vi "Weather Parse Test.vi"() -> ()   [LabVIEW 2020, in "CDM-Config.lvlib"] (continued)
\"Avoid\",\n                \"parameters\": {\n                    \"AWIPSidentifier\": [\n                        \"MWWCLE\"\n                    ],\n                    \"WMOidentifier\": [\n                        \"WHUS71 KCLE 031442\"\n                    ],\n                    \"NWSheadline\": [\n                        \"SMALL CRAFT ADVISORY REMAINS IN EFFECT UNTIL 7 PM EST THURSDAY... ...LOW WATER ADVISORY REMAINS IN EFFECT UNTIL 10 PM EST THIS EVENING\"\n                    ],\n                    \"BLOCKCHANNEL\": [\n                        \"EAS\",\n                        \"NWEM\",\n                        \"CMAS\"\n                    ],\n                    \"VTEC\": [\n                        \"/O.CON.KCLE.SC.Y.0072.000000T0000Z-251205T0000Z/\"\n                    ],\n                    \"eventEndingTime\": [\n                        \"2025-12-04T19:00:00-05:00\"\n                    ],\n                    \"expiredReferences\": [\n                        \"w-nws.webmaster@noaa.gov,urn:oid:2.49.0.1.840.0.0c886383843e06dfcc6ba0a1dce77e56032b6216.002.1,2025-12-02T21:44:00-05:00\"\n                    ]\n                },\n                \"scope\": \"Public\",\n                \"code\": \"IPAWSv1.0\",\n                \"language\": \"en-US\",\n                \"web\": \"http://www.weather.gov\",\n                \"eventCode\": {\n                    \"SAME\": [\n                        \"NWS\"\n                    ],\n                    \"NationalWeatherService\": [\n                        \"SCY\"\n                    ]\n                }\n            }\n        },\n        {\n            \"id\": \"https://api.weather.gov/alerts/urn:oid:2.49.0.1.840.0.459139686b06dc7377a32ee0b95bac1f049c2e93.001.1\",\n            \"type\": \"Feature\",\n            \"geometry\": null,\n            \"properties\": {\n                \"@id\": \"https://api.weather.gov/alerts/urn:oid:2.49.0.1.840.0.459139686b06dc7377a32ee0b95bac1f049c2e93.001.1\",\n                \"@type\": \"wx:Alert\",\n                \"id\": \"urn:oid:2.49.0.1.840.0.459139686b06dc7377a32ee0b95bac1f049c2e93.001.1\",\n                \"areaDesc\": \"Eastern Glacier, Western Toole, and Central Pondera; Southern High Plains; Eastern Pondera and Eastern Teton; Cascade County below 5000ft; Judith Basin County and Judith Gap; Gates of the Mountains\",\n                \"geocode\": {\n                    \"SAME\": [\n                        \"030035\",\n                        \"030073\",\n                        \"030101\",\n                        \"030049\",\n                        \"030099\",\n                        \"030013\",\n                        \"030045\",\n                        \"030027\"\n                    ],\n                    \"UGC\": [\n                        \"MTZ303\",\n                        \"MTZ308\",\n                        \"MTZ309\",\n                        \"MTZ312\",\n                        \"MTZ313\",\n                        \"MTZ316\"\n                    ]\n                },\n                \"affectedZones\": [\n                    \"https://api.weather.gov/zones/forecast/MTZ303\",\n                    \"https://api.weather.gov/zones/forecast/MTZ308\",\n                    \"https://api.weather.gov/zones/forecast/MTZ309\",\n                    \"https://api.weather.gov/zones/forecast/MTZ312\",\n                    \"https://api.weather.gov/zones/forecast/MTZ313\",\n                    \"https://api.weather.gov/zones/forecast/MTZ316\"\n                ],\n                \"references\": [],\n                \"sent\": \"2025-12-03T07:40:00-07:00\",\n                \"effective\": \"2025-12-03T07:40:00-07:00\",\n                \"onset\": \"2025-12-03T07:40:00-07:00\",\n                \"expires\": \"2025-12-03T10:00:00-07:00\",\n                \"ends\": null,\n                \"status\": \"Actual\",\n                \"messageType\": \"Alert\",\n                \"category\": \"Met\",\n                \"severity\": \"Moderate\",\n                \"certainty\": \"Observed\",\n                \"urgency\": \"Expected\",\n                \"event\": \"Special Weather Statement\",\n                \"sender\": \"w-nws.webmaster@noaa.gov\",\n                \"senderName\": \"NWS Great Falls MT\",\n                \"headline\": \"Special Weather Statement issued December 3 at 7:40AM MST by NWS Great Falls MT\",\n                \"description\": \"Patchy dense freezing fog is possible across portions of north-\\ncentral Montana this morning. Reduced visibility, in combination\\nwith icy roads, may make travel difficult at times. Motorists\\nshould be prepared for sudden changes in visibility and road\\nconditions.\",\n                \"instruction\": null,\n                \"response\": \"Execute\",\n                \"parameters\": {\n                    \"AWIPSidentifier\": [\n                        \"SPSTFX\"\n                    ],\n                    \"WMOidentifier\": [\n                        \"WWUS85 KTFX 031440\"\n                    ],\n                    \"BLOCKCHANNEL\": [\n                        \"EAS\",\n                        \"NWEM\",\n                        \"CMAS\"\n                    ],\n                    \"EAS-ORG\": [\n                        \"WXR\"\n                    ]\n                },\n                \"scope\": \"Public\",\n                \"code\": \"IPAWSv1.0\",\n                \"language\": \"en-US\",\n                \"web\": \"http://www.weather.gov\",\n                \"eventCode\": {\n                    \"SAME\": [\n                        \"SPS\"\n                    ],\n                    \"NationalWeatherService\": [\n                        \"SPS\"\n                    ]\n                }\n            }\n        },\n        {\n            \"id\": \"https://api.weather.gov/alerts/urn:oid:2.49.0.1.840.0.d9de63c9900d21dbac134cf2fe7828d3f5276171.002.2\",\n            \"type\": \"Feature\",\n            \"geometry\": null,\n            \"properties\": {\n                \"@id\": \"https://api.weather.gov/alerts/urn:oid:2.49.0.1.840.0.d9de63c9900d21dbac134cf2fe7828d3f5276171.002.2\",\n                \"@type\": \"wx:Alert\",\n                \"id\": \"urn:oid:2.49.0.1.840.0.d9de63c9900d21dbac134cf2fe7828d3f5276171.002.2\",\n                \"areaDesc\": \"Penobscot Bay; Casco Bay\",\n                \"geocode\": {\n                    \"SAME\": [\n                        \"073151\",\n                        \"073153\"\n                    ],\n                    \"UGC\": [\n                        \"ANZ151\",\n                        \"ANZ153\"\n                    ]\n                },\n                \"affectedZones\": [\n                    \"https://api.weather.gov/zones/forecast/ANZ151\",\n                    \"https://api.weather.gov/zones/forecast/ANZ153\"\n                ],\n                \"references\": [],\n                \"sent\": \"2025-12-03T09:35:00-05:00\",\n                \"effective\": \"2025-12-03T09:35:00-05:00\",\n                \"onset\": \"2025-12-04T13:00:00-05:00\",\n                \"expires\": \"2025-12-03T23:45:00-05:00\",\n                \"ends\": \"2025-12-05T07:00:00-05:00\",\n                \"status\": \"Actual\",\n                \"messageType\": \"Alert\",\n                \"category\": \"Met\",\n                \"severity\": \"Minor\",\n                \"certainty\": \"Likely\",\n                \"urgency\": \"Expected\",\n                \"event\": \"Small Craft Advisory\",\n                \"sender\": \"w-nws.webmaster@noaa.gov\",\n                \"senderName\": \"NWS Gray ME\",\n                \"headline\": \"Small Craft Advisory issued December 3 at 9:35AM EST until December 5 at 7:00AM EST by NWS Gray ME\",\n                \"description\": \"* WHAT...Northwest winds 15 to 25 kt with gusts up to 30 kt and\\nseas 2 to 5 ft expected.\\n\\n* WHERE...Penobscot Bay and Casco Bay.\\n\\n* WHEN...From 1 PM Thursday to 7 AM EST Friday.\\n\\n* IMPACTS...Conditions will be hazardous to small craft.\",\n                \"instruction\": \"Inexperienced mariners, especially those operating smaller\\nvessels, should avoid navigating in hazardous conditions.\",\n                \"response\": \"Avoid\",\n                \"parameters\": {\n                    \"AWIPSidentifier\": [\n                        \"MWWGYX\"\n                    ],\n                    \"WMOidentifier\": [\n                        \"WHUS71 KGYX 031435\"\n                    ],\n                    \"NWSheadline\": [\n                        \"SMALL CRAFT ADVISORY IN EFFECT FROM 1 PM THURSDAY TO 7 AM EST FRIDAY... ...SMALL CRAFT ADVISORY IS CANCELLED\"\n                    ],\n                    \"BLOCKCHANNEL\": [\n                        \"EAS\",\n                        \"NWEM\",\n                        \"CMAS\"\n                    ],\n                    \"VTEC\": [\n                        \"/O.NEW.KGYX.SC.Y.0091.251204T1800Z-251205T1200Z/\"\n                    ],\n                    \"eventEndingTime\": [\n                        \"2025-12-05T07:00:00-05:00\"\n                    ]\n                },\n                \"scope\": \"Public\",\n                \"code\": \"IPAWSv1.0\",\n                \"language\": \"en-US\",\n                \"web\": \"http://www.weather.gov\",\n                \"eventCode\": {\n                    \"SAME\": [\n                        \"NWS\"\n                    ],\n                    \"NationalWeatherService\": [\n                        \"SCY\"\n                    ]\n                }\n            }\n        },\n        {\n            \"id\": \"https://api.weather.gov/alerts/urn:oid:2.49.0.1.840.0.d9de63c9900d21dbac134cf2fe7828d3f5276171.001.2\",\n            \"type\": \"Feature\",\n            \"geometry\": null,\n            \"properties\": {\n                \"@id\": \"https://api.weather.gov/alerts/urn:oid:2.49.0.1.840.0.d9de63c9900d21dbac134cf2fe7828d3f5276171.001.2\",\n                \"@type\": \"wx:Alert\",\n                \"id\": \"urn:oid:2.49.0.1.840.0.d9de63c9900d21dbac134cf2fe7828d3f5276171.001.2\",\n                \"areaDesc\": \"Coastal Waters from Stonington, ME to Port Clyde, ME out 25 NM; Coastal Waters from Port Clyde, ME to Cape Elizabeth, ME out 25 NM; Coastal Waters from Cape Elizabeth, ME to Merrimack River, MA out 25 NM\",\n                \"geocode\": {\n                    \"SAME\": [\n                        \"073150\",\n                        \"073152\",\n                        \"073154\"\n                    ],\n                    \"UGC\": [\n                        \"ANZ150\",\n                        \"ANZ152\",\n                        \"ANZ154\"\n                    ]\n                },\n                \"affectedZones\": [\n                    \"https://api.weather.gov/zones/forecast/ANZ150\",\n                    \"https://api.weather.gov/zones/forecast/ANZ152\",\n                    \"https://api.weather.gov/zones/forecast/ANZ154\"\n                ],\n                \"references\": [],\n                \"sent\": \"2025-12-03T09:35:00-05:00\",\n                \"effective\": \"2025-12-03T09:35:00-05:00\",\n                \"onset\": \"2025-12-04T15:00:00-05:00\",\n                \"expires\": \"2025-12-03T23:45:00-05:00\",\n                \"ends\": \"2025-12-05T00:00:00-05:00\",\n                \"status\": \"Actual\",\n                \"messageType\": \"Alert\",\n                \"category\": \"Met\",\n                \"severity\": \"Moderate\",\n                \"certainty\": \"Likely\",\n                \"urgency\": \"Expected\",\n                \"event\": \"Gale Warning\",\n                \"sender\": \"w-nws.webmaster@noaa.gov\",\n                \"senderName\": \"NWS Gray ME\",\n                \"headline\": \"Gale Warning issued December 3 at 9:35AM EST until December 5 at 12:00AM EST by NWS Gray ME\",\n                \"description\": \"* WHAT...Northwest winds 20 to 30 kt with gusts up to 40 kt and\\nseas 5 to 8 ft expected.\\n\\n* WHERE...Coastal Waters from Stonington, ME to Port Clyde, ME\\nout 25 NM, Coastal Waters from Port Clyde, ME to Cape\\nElizabeth, ME out 25 NM and Coastal Waters from Cape\\nElizabeth, ME to Merrimack River, MA out 25 NM.\\n\\n* WHEN...From 3 PM Thursday to midnight EST Thursday night.\\n\\n* IMPACTS...Strong winds will cause hazardous seas which could\\ncapsize or damage vessels and reduce visibility.\",\n                \"instruction\": \"Mariners should alter plans to avoid these hazardous conditions.\\nRemain in port, seek safe harbor, alter course, and/or secure the\\nvessel for severe conditions.\",\n                \"response\": \"Avoid\",\n                \"parameters\": {\n                    \"AWIPSidentifier\": [\n                        \"MWWGYX\"\n                    ],\n                    \"WMOidentifier\": [\n                        \"WHUS71 KGYX 031435\"\n                    ],\n                    \"NWSheadline\": [\n                        \"GALE WARNING IN EFFECT FROM 3 PM THURSDAY TO MIDNIGHT EST THURSDAY NIGHT... ...GALE WARNING IS CANCELLED\"\n                    ],\n                    \"BLOCKCHANNEL\": [\n                        \"EAS\",\n                        \"NWEM\",\n                        \"CMAS\"\n                    ],\n                    \"VTEC\": [\n                        \"/O.NEW.KGYX.GL.W.0036.251204T2000Z-251205T0500Z/\"\n                    ],\n                    \"eventEndingTime\": [\n                        \"2025-12-05T00:00:00-05:00\"\n                    ]\n                },\n                \"scope\": \"Public\",\n                \"code\": \"IPAWSv1.0\",\n                \"language\": \"en-US\",\n                \"web\": \"http://www.weather.gov\",\n                \"eventCode\": {\n                    \"SAME\": [\n                        \"NWS\"\n                    ],\n                    \"NationalWeatherService\": [\n                        \"GLW\"\n                    ]\n                }\n            }\n        },\n        {\n            \"id\": \"https://api.weather.gov/alerts/urn:oid:2.49.0.1.840.0.168ce73ea8a3865ae0fef26c6698f44454ec2ed2.001.1\",\n            \"type\": \"Feature\",\n            \"geometry\": null,\n            \"properties\": {\n                \"@id\": \"https://api.weather.gov/alerts/urn:oid:2.49.0.1.840.0.168ce73ea8a3865ae0fef26c6698f44454ec2ed2.001.1\",\n                \"@type\": \"wx:Alert\",\n                \"id\": \"urn:oid:2.49.0.1.840.0.168ce73ea8a3865ae0fef26c6698f44454ec2ed2.001.1\",\n                \"areaDesc\": \"St Joseph to South Haven MI; South Haven to Holland MI; Holland to Grand Haven MI; Grand Haven to Whitehall MI; Whitehall to Pentwater MI; Pentwater to Manistee MI\",\n                \"geocode\": {\n                    \"SAME\": [\n                        \"092844\",\n                        \"092845\",\n                        \"092846\",\n                        \"092847\",\n                        \"092848\",\n                        \"092849\"\n                    ],\n                    \"UGC\": [\n                        \"LMZ844\",\n                        \"LMZ845\",\n                        \"LMZ846\",\n                        \"LMZ847\",\n                        \"LMZ848\",\n                        \"LMZ849\"\n                    ]\n                },\n                \"affectedZones\": [\n                    \"https://api.weather.gov/zones/forecast/LMZ844\",\n                    \"https://api.weather.gov/zones/forecast/LMZ845\",\n                    \"https://api.weather.gov/zones/forecast/LMZ846\",\n                    \"https://api.weather.gov/zones/forecast/LMZ847\",\n                    \"https://api.weather.gov/zones/forecast/LMZ848\",\n                    \"https://api.weather.gov/zones/forecast/LMZ849\"\n                ],\n                \"references\": [\n                    {\n                        \"@id\": \"https://api.weather.gov/alerts/urn:oid:2.49.0.1.840.0.7aaab00944e439757f97bf60c2973af97298ac0f.001.1\",\n                        \"identifier\": \"urn:oid:2.49.0.1.840.0.7aaab00944e439757f97bf60c2973af97298ac0f.001.1\",\n                        \"sender\": \"w-nws.webmaster@noaa.gov\",\n                        \"sent\": \"2025-12-03T03:29:00-05:00\"\n                    }\n                ],\n                \"sent\": \"2025-12-03T09:32:00-05:00\",\n                \"effective\": \"2025-12-03T09:32:00-05:00\",\n                \"onset\": \"2025-12-03T09:32:00-05:00\",\n                \"expires\": \"2025-12-03T17:45:00-05:00\",\n                \"ends\": \"2025-12-04T19:00:00-05:00\",\n                \"status\": \"Actual\",\n                \"messageType\": \"Update\",\n                \"category\": \"Met\",\n                \"severity\": \"Minor\",\n                \"certainty\": \"Likely\",\n                \"urgency\": \"Expected\",\n                \"event\": \"Small Craft Advisory\",\n                \"sender\": \"w-nws.webmaster@noaa.gov\",\n                \"senderName\": \"NWS Grand Rapids MI\",\n                \"headline\": \"Small Craft Advisory issued December 3 at 9:32AM EST until December 4 at 7:00PM EST by NWS Grand Rapids MI\",\n                \"description\": \"* WHAT...Northwest winds 15 to 25 knots with gusts up to 30\\nknots and waves 6 to 9 feet.\\n\\n* WHERE...St Joseph to Manistee.\\n\\n* WHEN...Until 7 PM EST Thursday.\\n\\n* IMPACTS...Conditions will be hazardous to small craft.\",\n                \"instruction\": \"Inexperienced mariners, especially those operating smaller\\nvessels, should avoid navigating in hazardous conditions.\",\n                \"response\": \"Avoid\",\n                \"parameters\": {\n                    \"AWIPSidentifier\": [\n                        \"MWWGRR\"\n                    ],\n                    \"WMOidentifier\": [\n                        \"WHUS73 KGRR 031432\"\n                    ],\n                    \"NWSheadline\": [\n                        \"SMALL CRAFT ADVISORY REMAINS IN EFFECT UNTIL 7 PM EST THURSDAY\"\n                    ],\n                    \"BLOCKCHANNEL\": [\n                        \"EAS\",\n                        \"NWEM\",\n                        \"CMAS\"\n                    ],\n                    \"VTEC\": [\n                        \"/O.CON.KGRR.SC.Y.0105.000000T0000Z-251205T0000Z/\"\n                    ],\n                    \"eventEndingTime\": [\n                        \"2025-12-04T19:00:00-05:00\"\n                    ],\n                    \"expiredReferences\": [\n                        \"w-nws.webmaster@noaa.gov,urn:oid:2.49.0.1.840.0.d51c6ec7dcdb20057f5ceabbc87dc36d93f53d9d.001.1,2025-12-02T22:57:00-05:00 w-nws.webmaster@noaa.gov,urn:oid:2.49.0.1.840.0.37bcc3e39a4ce8355e137c1eb2919fee8e6cd4f1.001.1,2025-12-02T15:51:00-05:00 w-nws.webmaster@noaa.gov,urn:oid:2.49.0.1.840.0.c3d7b241827877fcb2062e6796861e8d3cd92a63.001.1,2025-12-02T09:46:00-05:00 w-nws.webmaster@noaa.gov,urn:oid:2.49.0.1.840.0.67f802fa2a1d1ee3a1aa8fcbfdeb00afe1d79cbe.001.1,2025-12-02T03:07:00-05:00\"\n                    ]\n                },\n                \"scope\": \"Public\",\n                \"code\": \"IPAWSv1.0\",\n                \"language\": \"en-US\",\n                \"web\": \"http://www.weather.gov\",\n                \"eventCode\": {\n                    \"SAME\": [\n                        \"NWS\"\n                    ],\n                    \"NationalWeatherService\": [\n                        \"SCY\"\n                    ]\n                }\n            }\n        },\n        {\n            \"id\": \"https://api.weather.gov/alerts/urn:oid:2.49.0.1.840.0.1012c94d5f34968dad73e0ece48bd6552b3e5229.005.1\",\n            \"type\": \"Feature\",\n            \"geometry\": null,\n            \"properties\": {\n                \"@id\": \"https://api.weather.gov/alerts/urn:oid:2.49.0.1.840.0.1012c94d5f34968dad73e0ece48bd6552b3e5229.005.1\",\n                \"@type\": \"wx:Alert\",\n                \"id\": \"urn:oid:2.49.0.1.840.0.1012c94d5f34968dad73e0ece48bd6552b3e5229.005.1\",\n                \"areaDesc\": \"Boston Harbor; Narragansett Bay\",\n                \"geocode\": {\n                    \"SAME\": [\n                        \"073230\",\n                        \"073236\"\n                    ],\n                    \"UGC\": [\n                        \"ANZ230\",\n                        \"ANZ236\"\n                    ]\n                },\n                \"affectedZones\": [\n                    \"https://api.weather.gov/zones/forecast/ANZ230\",\n                    \"https://api.weather.gov/zones/forecast/ANZ236\"\n                ],\n                \"references\": [],\n                \"sent\": \"2025-12-03T09:03:00-05:00\",\n                \"effective\": \"2025-12-03T09:03:00-05:00\",\n                \"onset\": \"2025-12-04T13:00:00-05:00\",\n                \"expires\": \"2025-12-03T22:15:00-05:00\",\n                \"ends\": \"2025-12-05T01:00:00-05:00\",\n                \"status\": \"Actual\",\n                \"messageType\": \"Alert\",\n                \"category\": \"Met\",\n                \"severity\": \"Moderate\",\n                \"certainty\": \"Possible\",\n                \"urgency\": \"Future\",\n                \"event\": \"Gale Watch\",\n                \"sender\": \"w-nws.webmaster@noaa.gov\",\n                \"senderName\": \"NWS Boston/Norton MA\",\n                \"headline\": \"Gale Watch issued December 3 at 9:03AM EST until December 5 at 1:00AM EST by NWS Boston/Norton MA\",\n                \"description\": \"* WHAT...Northwest winds 15 to 25 kt with gusts up to 35 kt and\\nwaves 2 to 3 feet possible.\\n\\n* WHERE...In Massachusetts coastal waters, Boston Harbor. In\\nRhode Island coastal waters, Narragansett Bay.\\n\\n* WHEN...From Thursday afternoon through late Thursday night.\\n\\n* IMPACTS...Strong winds can cause hazardous waves which could\\ncapsize or damage vessels and reduce visibility.\",\n                \"instruction\": \"Mariners should consider altering plans to avoid possible\\nhazardous conditions.  Remain in port, seek safe harbor, alter\\ncourse, and/or secure the vessel for severe wind and seas.\",\n                \"response\": \"Prepare\",\n                \"parameters\": {\n                    \"AWIPSidentifier\": [\n                        \"MWWBOX\"\n                    ],\n                    \"WMOidentifier\": [\n                        \"WHUS71 KBOX 031403\"\n                    ],\n                    \"NWSheadline\": [\n                        \"GALE WATCH IN EFFECT FROM THURSDAY AFTERNOON THROUGH LATE THURSDAY NIGHT\"\n                    ],\n                    \"BLOCKCHANNEL\": [\n                        \"EAS\",\n                        \"NWEM\",\n                        \"CMAS\"\n                    ],\n                    \"VTEC\": [\n                        \"/O.NEW.KBOX.GL.A.0024.251204T1800Z-251205T0600Z/\"\n                    ],\n                    \"eventEndingTime\": [\n                        \"2025-12-05T01:00:00-05:00\"\n                    ]\n                },\n                \"scope\": \"Public\",\n                \"code\": \"IPAWSv1.0\",\n                \"language\": \"en-US\",\n                \"web\": \"http://www.weather.gov\",\n                \"eventCode\": {\n                    \"SAME\": [\n                        \"NWS\"\n                    ],\n                    \"NationalWeatherService\": [\n                        \"GLA\"\n                    ]\n                }\n            }\n        },\n        {\n            \"id\": \"https://api.weather.gov/alerts/urn:oid:2.49.0.1.840.0.1012c94d5f34968dad73e0ece48bd6552b3e5229.001.3\",\n            \"type\": \"Feature\",\n            \"geometry\": null,\n            \"properties\": {\n                \"@id\": \"https://api.weather.gov/alerts/urn:oid:2.49.0.1.840.0.1012c94d5f34968dad73e0ece48bd6552b3e5229.001.3\",\n                \"@type\": \"wx:Alert\",\n                \"id\": \"urn:oid:2.49.0.1.840.0.1012c94d5f34968dad73e0ece48bd6552b3e5229.001.3\",\n                \"areaDesc\": \"Coastal waters east of Ipswich Bay and the Stellwagen Bank National Marine Sanctuary; Coastal waters from Provincetown MA to Chatham MA to Nantucket MA out 20 nm; Coastal Waters extending out to 25 nm South of Marthas Vineyard and Nantucket\",\n                \"geocode\": {\n                    \"SAME\": [\n                        \"073250\",\n                        \"073254\",\n                        \"073255\"\n                    ],\n                    \"UGC\": [\n                        \"ANZ250\",\n                        \"ANZ254\",\n                        \"ANZ255\"\n                    ]\n                },\n                \"affectedZones\": [\n                    \"https://api.weather.gov/zones/forecast/ANZ250\",\n                    \"https://api.weather.gov/zones/forecast/ANZ254\",\n                    \"https://api.weather.gov/zones/forecast/ANZ255\"\n                ],\n                \"references\": [],\n                \"sent\": \"2025-12-03T09:03:00-05:00\",\n                \"effective\": \"2025-12-03T09:03:00-05:00\",\n                \"onset\": \"2025-12-04T13:00:00-05:00\",\n                \"expires\": \"2025-12-03T22:15:00-05:00\",\n                \"ends\": \"2025-12-05T04:00:00-05:00\",\n                \"status\": \"Actual\",\n                \"messageType\": \"Alert\",\n                \"category\": \"Met\",\n                \"severity\": \"Moderate\",\n                \"certainty\": \"Likely\",\n                \"urgency\": \"Expected\",\n                \"event\": \"Gale Warning\",\n                \"sender\": \"w-nws.webmaster@noaa.gov\",\n                \"senderName\": \"NWS Boston/Norton MA\",\n                \"headline\": \"Gale Warning issued December 3 at 9:03AM EST until December 5 at 4:00AM EST by NWS Boston/Norton MA\",\n                \"description\": \"* WHAT...Northwest winds 25 to 35 kt with gusts up to 40 kt and\\nseas 5 to 8 feet expected.\\n\\n* WHERE...Coastal waters east of Ipswich Bay and the Stellwagen\\nBank National Marine Sanctuary, Coastal waters from\\nProvincetown MA to Chatham MA to Nantucket MA out 20 nm and\\nCoastal Waters extending out to 25 nm South of Marthas\\nVineyard and Nantucket.\\n\\n* WHEN...From 1 PM Thursday to 4 AM EST Friday.\\n\\n* IMPACTS...Strong winds will cause hazardous seas which could\\ncapsize or damage vessels and reduce visibility.\",\n                \"instruction\": \"Mariners should alter plans to avoid these hazardous conditions.\\nRemain in port, seek safe harbor, alter course, and/or secure the\\nvessel for hazardous conditions.\",\n                \"response\": \"Avoid\",\n                \"parameters\": {\n                    \"AWIPSidentifier\": [\n                        \"MWWBOX\"\n                    ],\n                    \"WMOidentifier\": [\n                        \"WHUS71 KBOX 031403\"\n                    ],\n                    \"NWSheadline\": [\n                        \"GALE WARNING IN EFFECT FROM 1 PM THURSDAY TO 4 AM EST FRIDAY\"\n                    ],\n                    \"BLOCKCHANNEL\": [\n                        \"EAS\",\n                        \"NWEM\",\n                        \"CMAS\"\n                    ],\n                    \"VTEC\": [\n                        \"/O.NEW.KBOX.GL.W.0040.251204T1800Z-251205T0900Z/\"\n                    ],\n                    \"eventEndingTime\": [\n                        \"2025-12-05T04:00:00-05:00\"\n                    ]\n                },\n                \"scope\": \"Public\",\n                \"code\": \"IPAWSv1.0\",\n                \"language\": \"en-US\",\n                \"web\": \"http://www.weather.gov\",\n                \"eventCode\": {\n                    \"SAME\": [\n                        \"NWS\"\n                    ],\n                    \"NationalWeatherService\": [\n                        \"GLW\"\n                    ]\n                }\n            }\n        },\n        {\n            \"id\": \"https://api.weather.gov/alerts/urn:oid:2.49.0.1.840.0.1012c94d5f34968dad73e0ece48bd6552b3e5229.003.3\",\n            \"type\": \"Feature\",\n            \"geometry\": null,\n            \"properties\": {\n                \"@id\": \"https://api.weather.gov/alerts/urn:oid:2.49.0.1.840.0.1012c94d5f34968dad73e0ece48bd6552b3e5229.003.3\",\n                \"@type\": \"wx:Alert\",\n                \"id\": \"urn:oid:2.49.0.1.840.0.1012c94d5f34968dad73e0ece48bd6552b3e5229.003.3\",\n                \"areaDesc\": \"Coastal Waters from Montauk NY to Marthas Vineyard extending out to 20 nm South of Block Island\",\n                \"geocode\": {\n                    \"SAME\": [\n                        \"073256\"\n                    ],\n                    \"UGC\": [\n                        \"ANZ256\"\n                    ]\n                },\n                \"affectedZones\": [\n                    \"https://api.weather.gov/zones/forecast/ANZ256\"\n                ],\n                \"references\": [],\n                \"sent\": \"2025-12-03T09:03:00-05:00\",\n                \"effective\": \"2025-12-03T09:03:00-05:00\",\n                \"onset\": \"2025-12-04T13:00:00-05:00\",\n                \"expires\": \"2025-12-03T22:15:00-05:00\",\n                \"ends\": \"2025-12-05T04:00:00-05:00\",\n                \"status\": \"Actual\",\n                \"messageType\": \"Alert\",\n                \"category\": \"Met\",\n                \"severity\": \"Moderate\",\n                \"certainty\": \"Likely\",\n                \"urgency\": \"Expected\",\n                \"event\": \"Gale Warning\",\n                \"sender\": \"w-nws.webmaster@noaa.gov\",\n                \"senderName\": \"NWS Boston/Norton MA\",\n                \"headline\": \"Gale Warning issued December 3 at 9:03AM EST until December 5 at 4:00AM EST by NWS Boston/Norton MA\",\n                \"description\": \"* WHAT...Northwest winds 20 to 30 kt with gusts up to 40 kt and\\nseas 5 to 8 feet expected.\\n\\n* WHERE...Coastal Waters from Montauk NY to Marthas Vineyard\\nextending out to 20 nm South of Block Island.\\n\\n* WHEN...From 1 PM Thursday to 4 AM EST Friday.\\n\\n* IMPACTS...Strong winds will cause hazardous seas which could\\ncapsize or damage vessels and reduce visibility.\",\n                \"instruction\": \"Mariners should alter plans to avoid these hazardous conditions.\\nRemain in port, seek safe harbor, alter course, and/or secure the\\nvessel for hazardous conditions.\",\n                \"response\": \"Avoid\",\n                \"parameters\": {\n                    \"AWIPSidentifier\": [\n                        \"MWWBOX\"\n                    ],\n                    \"WMOidentifier\": [\n                        \"WHUS71 KBOX 031403\"\n                    ],\n                    \"NWSheadline\": [\n                        \"GALE WARNING IN EFFECT FROM 1 PM THURSDAY TO 4 AM EST FRIDAY\"\n                    ],\n                    \"BLOCKCHANNEL\": [\n                        \"EAS\",\n                        \"NWEM\",\n                        \"CMAS\"\n                    ],\n                    \"VTEC\": [\n                        \"/O.NEW.KBOX.GL.W.0040.251204T1800Z-251205T0900Z/\"\n                    ],\n                    \"eventEndingTime\": [\n                        \"2025-12-05T04:00:00-05:00\"\n                    ]\n                },\n                \"scope\": \"Public\",\n                \"code\": \"IPAWSv1.0\",\n                \"language\": \"en-US\",\n                \"web\": \"http://www.weather.gov\",\n                \"eventCode\": {\n                    \"SAME\": [\n                        \"NWS\"\n                    ],\n                    \"NationalWeatherService\": [\n                        \"GLW\"\n                    ]\n                }\n            }\n        },\n        {\n            \"id\": \"https://api.weather.gov/alerts/urn:oid:2.49.0.1.840.0.1012c94d5f34968dad73e0ece48bd6552b3e5229.002.3\",\n            \"type\": \"Feature\",\n            \"geometry\": null,\n            \"properties\": {\n                \"@id\": \"https://api.weather.gov/alerts/urn:oid:2.49.0.1.840.0.1012c94d5f34968dad73e0ece48bd6552b3e5229.002.3\",\n                \"@type\": \"wx:Alert\",\n                \"id\": \"urn:oid:2.49.0.1.840.0.1012c94d5f34968dad73e0ece48bd6552b3e5229.002.3\",\n                \"areaDesc\": \"Cape Cod Bay; Nantucket Sound; Massachusetts Bay and Ipswich Bay\",\n                \"geocode\": {\n                    \"SAME\": [\n                        \"073231\",\n                        \"073232\",\n                        \"073251\"\n                    ],\n                    \"UGC\": [\n                        \"ANZ231\",\n                        \"ANZ232\",\n                        \"ANZ251\"\n                    ]\n                },\n                \"affectedZones\": [\n                    \"https://api.weather.gov/zones/forecast/ANZ231\",\n                    \"https://api.weather.gov/zones/forecast/ANZ232\",\n                    \"https://api.weather.gov/zones/forecast/ANZ251\"\n                ],\n                \"references\": [],\n                \"sent\": \"2025-12-03T09:03:00-05:00\",\n                \"effective\": \"2025-12-03T09:03:00-05:00\",\n                \"onset\": \"2025-12-04T13:00:00-05:00\",\n                \"expires\": \"2025-12-03T22:15:00-05:00\",\n                \"ends\": \"2025-12-05T04:00:00-05:00\",\n                \"status\": \"Actual\",\n                \"messageType\": \"Alert\",\n                \"category\": \"Met\",\n                \"severity\": \"Moderate\",\n                \"certainty\": \"Likely\",\n                \"urgency\": \"Expected\",\n                \"event\": \"Gale Warning\",\n                \"sender\": \"w-nws.webmaster@noaa.gov\",\n                \"senderName\": \"NWS Boston/Norton MA\",\n                \"headline\": \"Gale Warning issued December 3 at 9:03AM EST until December 5 at 4:00AM EST by NWS Boston/Norton MA\",\n                \"description\": \"* WHAT...Northwest winds 20 to 30 kt with gusts up to 40 kt and\\nseas 3 to 5 feet expected.\\n\\n* WHERE...Cape Cod Bay, Nantucket Sound and Massachusetts Bay\\nand Ipswich Bay.\\n\\n* WHEN...From 1 PM Thursday to 4 AM EST Friday.\\n\\n* IMPACTS...Strong winds will cause hazardous seas which could\\ncapsize or damage vessels and reduce visibility.\",\n                \"instruction\": \"Mariners should alter plans to avoid these hazardous conditions.\\nRemain in port, seek safe harbor, alter course, and/or secure the\\nvessel for hazardous conditions.\",\n                \"response\": \"Avoid\",\n                \"parameters\": {\n                    \"AWIPSidentifier\": [\n                        \"MWWBOX\"\n                    ],\n                    \"WMOidentifier\": [\n                        \"WHUS71 KBOX 031403\"\n                    ],\n                    \"NWSheadline\": [\n                        \"GALE WARNING IN EFFECT FROM 1 PM THURSDAY TO 4 AM EST FRIDAY\"\n                    ],\n                    \"BLOCKCHANNEL\": [\n                        \"EAS\",\n                        \"NWEM\",\n                        \"CMAS\"\n                    ],\n                    \"VTEC\": [\n                        \"/O.NEW.KBOX.GL.W.0040.251204T1800Z-251205T0900Z/\"\n                    ],\n                    \"eventEndingTime\": [\n                        \"2025-12-05T04:00:00-05:00\"\n                    ]\n                },\n                \"scope\": \"Public\",\n                \"code\": \"IPAWSv1.0\",\n                \"language\": \"en-US\",\n                \"web\": \"http://www.weather.gov\",\n                \"eventCode\": {\n                    \"SAME\": [\n                        \"NWS\"\n                    ],\n                    \"NationalWeatherService\": [\n                        \"GLW\"\n                    ]\n                }\n            }\n        },\n        {\n            \"id\": \"https://api.weather.gov/alerts/urn:oid:2.49.0.1.840.0.1012c94d5f34968dad73e0ece48bd6552b3e5229.004.2\",\n            \"type\": \"Feature\",\n            \"geometry\": null,\n            \"properties\": {\n                \"@id\": \"https://api.weather.gov/alerts/urn:oid:2.49.0.1.840.0.1012c94d5f34968dad73e0ece48bd6552b3e5229.004.2\",\n                \"@type\": \"wx:Alert\",\n                \"id\": \"urn:oid:2.49.0.1.840.0.1012c94d5f34968dad73e0ece48bd6552b3e5229.004.2\",\n                \"areaDesc\": \"Vineyard Sound; Buzzards Bay; Rhode Island Sound; Block Island Sound\",\n                \"geocode\": {\n                    \"SAME\": [\n                        \"073233\",\n                        \"073234\",\n                        \"073235\",\n                        \"073237\"\n                    ],\n                    \"UGC\": [\n                        \"ANZ233\",\n                        \"ANZ234\",\n                        \"ANZ235\",\n                        \"ANZ237\"\n                    ]\n                },\n                \"affectedZones\": [\n                    \"https://api.weather.gov/zones/forecast/ANZ233\",\n                    \"https://api.weather.gov/zones/forecast/ANZ234\",\n                    \"https://api.weather.gov/zones/forecast/ANZ235\",\n                    \"https://api.weather.gov/zones/forecast/ANZ237\"\n                ],\n                \"references\": [],\n                \"sent\": \"2025-12-03T09:03:00-05:00\",\n                \"effective\": \"2025-12-03T09:03:00-05:00\",\n                \"onset\": \"2025-12-04T13:00:00-05:00\",\n                \"expires\": \"2025-12-03T22:15:00-05:00\",\n                \"ends\": \"2025-12-05T04:00:00-05:00\",\n                \"status\": \"Actual\",\n                \"messageType\": \"Alert\",\n                \"category\": \"Met\",\n                \"severity\": \"Moderate\",\n                \"certainty\": \"Likely\",\n                \"urgency\": \"Expected\",\n                \"event\": \"Gale Warning\",\n                \"sender\": \"w-nws.webmaster@noaa.gov\",\n                \"senderName\": \"NWS Boston/Norton MA\",\n                \"headline\": \"Gale Warning issued December 3 at 9:03AM EST until December 5 at 4:00AM EST by NWS Boston/Norton MA\",\n                \"description\": \"* WHAT...Northwest winds 15 to 25 kt with gusts up to 40 kt and\\nseas 3 to 5 feet expected.\\n\\n* WHERE...In Massachusetts coastal waters, Vineyard Sound and\\nBuzzards Bay. In Rhode Island coastal waters, Rhode Island\\nSound and Block Island Sound.\\n\\n* WHEN...From 1 PM Thursday to 4 AM EST Friday.\\n\\n* IMPACTS...Strong winds will cause hazardous seas which could\\ncapsize or damage vessels and reduce visibility.\",\n                \"instruction\": \"Mariners should alter plans to avoid these hazardous conditions.\\nRemain in port, seek safe harbor, alter course, and/or secure the\\nvessel for hazardous conditions.\",\n                \"response\": \"Avoid\",\n                \"parameters\": {\n                    \"AWIPSidentifier\": [\n                        \"MWWBOX\"\n                    ],\n                    \"WMOidentifier\": [\n                        \"WHUS71 KBOX 031403\"\n                    ],\n                    \"NWSheadline\": [\n                        \"GALE WARNING IN EFFECT FROM 1 PM THURSDAY TO 4 AM EST FRIDAY\"\n                    ],\n                    \"BLOCKCHANNEL\": [\n                        \"EAS\",\n                        \"NWEM\",\n                        \"CMAS\"\n                    ],\n                    \"VTEC\": [\n                        \"/O.NEW.KBOX.GL.W.0040.251204T1800Z-251205T0900Z/\"\n                    ],\n                    \"eventEndingTime\": [\n                        \"2025-12-05T04:00:00-05:00\"\n                    ]\n                },\n                \"scope\": \"Public\",\n                \"code\": \"IPAWSv1.0\",\n                \"language\": \"en-US\",\n                \"web\": \"http://www.weather.gov\",\n                \"eventCode\": {\n                    \"SAME\": [\n                        \"NWS\"\n                    ],\n                    \"NationalWeatherService\": [\n                        \"GLW\"\n                    ]\n                }\n            }\n        },\n        {\n            \"id\": \"https://api.weather.gov/alerts/urn:oid:2.49.0.1.840.0.5a534255b812129f891a3e8033034b4dedccb030.001.1\",\n            \"type\": \"Feature\",\n            \"geometry\": null,\n            \"properties\": {\n                \"@id\": \"https://api.weather.gov/alerts/urn:oid:2.49.0.1.840.0.5a534255b812129f891a3e8033034b4dedccb030.001.1\",\n                \"@type\": \"wx:Alert\",\n                \"id\": \"urn:oid:2.49.0.1.840.0.5a534255b812129f891a3e8033034b4dedccb030.001.1\",\n                \"areaDesc\": \"Kuskokwim Delta and Etolin Strait out to 15 NM; Kuskokwim Delta from 15 to 80 NM; North and West of Nunivak Island\",\n                \"geocode\": {\n                    \"SAME\": [\n                        \"058763\",\n                        \"058764\",\n                        \"058765\"\n                    ],\n                    \"UGC\": [\n                        \"PKZ763\",\n                        \"PKZ764\",\n                        \"PKZ765\"\n                    ]\n                },\n                \"affectedZones\": [\n                    \"https://api.weather.gov/zones/forecast/PKZ763\",\n                    \"https://api.weather.gov/zones/forecast/PKZ764\",\n                    \"https://api.weather.gov/zones/forecast/PKZ765\"\n                ],\n                \"references\": [],\n                \"sent\": \"2025-12-03T04:19:00-09:00\",\n                \"effective\": \"2025-12-03T04:19:00-09:00\",\n                \"onset\": \"2025-12-03T04:19:00-09:00\",\n                \"expires\": \"2025-12-03T17:00:00-09:00\",\n                \"ends\": null,\n                \"status\": \"Actual\",\n                \"messageType\": \"Alert\",\n                \"category\": \"Met\",\n                \"severity\": \"Minor\",\n                \"certainty\": \"Observed\",\n                \"urgency\": \"Expected\",\n                \"event\": \"Marine Weather Statement\",\n                \"sender\": \"w-nws.webmaster@noaa.gov\",\n                \"senderName\": \"NWS Anchorage AK\",\n                \"headline\": \"Marine Weather Statement issued December 3 at 4:19AM AKST by NWS Anchorage AK\",\n                \"description\": \"Northeasterly winds in combination with Arctic Air could lead to\\nextreme vessel icing at rates of 4 cm per hour or greater.\\n\\nAs colder air filters in from the Arctic over the weekend, winds\\nwill become gusty and northeasterly. These factors will cause\\nextreme freezing spray which will spread south and west from the\\nKuskokwim Delta. Heavy to extreme freezing spray will extend from\\nCape Newenham to north and west of Nunivak Island by Saturday. It\\nwill likely last through Tuesday.\\n\\nOperating a vessel in heavy to extreme freezing spray is\\nhazardous. Freezing spray may render mechanical and electronic\\ncomponents inoperable. Rapid ice accretion on decks and\\nsuperstructures may result in catastrophic loss of stability.\",\n                \"instruction\": null,\n                \"response\": \"Monitor\",\n                \"parameters\": {\n                    \"AWIPSidentifier\": [\n                        \"MWSAFC\"\n                    ],\n                    \"WMOidentifier\": [\n                        \"FZAK78 PAFC 031319\"\n                    ],\n                    \"NWSheadline\": [\n                        \"EXTREME VESSEL ICING POSSIBLE FROM NORHT AND WEST OF NUNIVAK ISLAND TO CAPE NEWENHAM SATURDAY THROUGH TUESDAY\"\n                    ],\n                    \"BLOCKCHANNEL\": [\n                        \"EAS\",\n                        \"NWEM\",\n                        \"CMAS\"\n                    ]\n                },\n                \"scope\": \"Public\",\n                \"code\": \"IPAWSv1.0\",\n                \"language\": \"en-US\",\n                \"web\": \"http://www.weather.gov\",\n                \"eventCode\": {\n                    \"SAME\": [\n                        \"NWS\"\n                    ],\n                    \"NationalWeatherService\": [\n                        \"MWS\"\n                    ]\n                }\n            }\n        },\n        {\n            \"id\": \"https://api.weather.gov/alerts/urn:oid:2.49.0.1.840.0.3fac73b358a1e250101ceb2ba749b5bee3a29f80.018.1\",\n            \"type\": \"Feature\",\n            \"geometry\": null,\n            \"properties\": {\n                \"@id\": \"https://api.weather.gov/alerts/urn:oid:2.49.0.1.840.0.3fac73b358a1e250101ceb2ba749b5bee3a29f80.018.1\",\n                \"@type\": \"wx:Alert\",\n                \"id\": \"urn:oid:2.49.0.1.840.0.3fac73b358a1e250101ceb2ba749b5bee3a29f80.018.1\",\n                \"areaDesc\": \"Marmot Island to Sitkinak out to 15 NM\",\n                \"geocode\": {\n                    \"SAME\": [\n                        \"058732\"\n                    ],\n                    \"UGC\": [\n                        \"PKZ732\"\n                    ]\n                },\n                \"affectedZones\": [\n                    \"https://api.weather.gov/zones/forecast/PKZ732\"\n                ],\n                \"references\": [],\n                \"sent\": \"2025-12-03T04:02:00-09:00\",\n                \"effective\": \"2025-12-03T04:02:00-09:00\",\n                \"onset\": \"2025-12-03T04:00:00-09:00\",\n                \"expires\": \"2025-12-03T16:30:00-09:00\",\n                \"ends\": \"2025-12-04T17:00:00-09:00\",\n                \"status\": \"Actual\",\n                \"messageType\": \"Alert\",\n                \"category\": \"Met\",\n                \"severity\": \"Minor\",\n                \"certainty\": \"Likely\",\n                \"urgency\": \"Expected\",\n                \"event\": \"Small Craft Advisory\",\n                \"sender\": \"w-nws.webmaster@noaa.gov\",\n                \"senderName\": \"NWS Anchorage AK\",\n                \"headline\": \"Small Craft Advisory issued December 3 at 4:02AM AKST until December 4 at 5:00PM AKST by NWS Anchorage AK\",\n                \"description\": \"Coastal Waters Forecast for the Northern Gulf of Alaska Coast\\nup to 100 nm out including Kodiak Island and Cook Inlet.\\n\\nWind forecasts reflect the predominant speed and direction\\nexpected. Sea forecasts represent an average of the highest\\none-third of the combined wind wave and swell height.\\n\\n.TODAY...S wind 20 kt. Seas 12 ft.\\n.TONIGHT...S wind 15 kt. Seas 10 ft.\\n.THU...SE wind 15 kt. Seas 9 ft.\\n.THU NIGHT...NE wind 15 kt. Seas 6 ft.\\n.FRI THROUGH SAT...NW wind 25 kt. Seas 8 ft.\\n.SUN...NW wind 20 kt. Seas 11 ft.\",\n                \"instruction\": null,\n                \"response\": \"Avoid\",\n                \"parameters\": {\n                    \"AWIPSidentifier\": [\n                        \"CWFAER\"\n                    ],\n                    \"WMOidentifier\": [\n                        \"FZAK51 PAFC 031302\"\n                    ],\n                    \"NWSheadline\": [\n                        \"SMALL CRAFT ADVISORY THROUGH THURSDAY\"\n                    ],\n                    \"BLOCKCHANNEL\": [\n                        \"EAS\",\n                        \"NWEM\",\n                        \"CMAS\"\n                    ],\n                    \"VTEC\": [\n                        \"/O.NEW.PAFC.SC.Y.9736.251203T1300Z-251205T0200Z/\"\n                    ],\n                    \"eventEndingTime\": [\n                        \"2025-12-04T17:00:00-09:00\"\n                    ]\n                },\n                \"scope\": \"Public\",\n                \"code\": \"IPAWSv1.0\",\n                \"language\": \"en-US\",\n                \"web\": \"http://www.weather.gov\",\n                \"eventCode\": {\n                    \"SAME\": [\n                        \"NWS\"\n                    ],\n                    \"NationalWeatherService\": [\n                        \"SCY\"\n                    ]\n                }\n            }\n        },\n        {\n            \"id\": \"https://api.weather.gov/alerts/urn:oid:2.49.0.1.840.0.3fac73b358a1e250101ceb2ba749b5bee3a29f80.022.1\",\n            \"type\": \"Feature\",\n            \"geometry\": null,\n            \"properties\": {\n                \"@id\": \"https://api.weather.gov/alerts/urn:oid:2.49.0.1.840.0.3fac73b358a1e250101ceb2ba749b5bee3a29f80.022.1\",\n                \"@type\": \"wx:Alert\",\n                \"id\": \"urn:oid:2.49.0.1.840.0.3fac73b358a1e250101ceb2ba749b5bee3a29f80.022.1\",\n                \"areaDesc\": \"Shelikof Strait\",\n                \"geocode\": {\n                    \"SAME\": [\n                        \"058738\"\n                    ],\n                    \"UGC\": [\n                        \"PKZ738\"\n                    ]\n                },\n                \"affectedZones\": [\n                    \"https://api.weather.gov/zones/forecast/PKZ738\"\n                ],\n                \"references\": [],\n                \"sent\": \"2025-12-03T04:02:00-09:00\",\n                \"effective\": \"2025-12-03T04:02:00-09:00\",\n                \"onset\": \"2025-12-03T05:00:00-09:00\",\n                \"expires\": \"2025-12-03T16:30:00-09:00\",\n                \"ends\": \"2025-12-03T17:00:00-09:00\",\n                \"status\": \"Actual\",\n                \"messageType\": \"Alert\",\n                \"category\": \"Met\",\n                \"severity\": \"Minor\",\n                \"certainty\": \"Likely\",\n                \"urgency\": \"Expected\",\n                \"event\": \"Small Craft Advisory\",\n                \"sender\": \"w-nws.webmaster@noaa.gov\",\n                \"senderName\": \"NWS Anchorage AK\",\n                \"headline\": \"Small Craft Advisory issued December 3 at 4:02AM AKST until December 3 at 5:00PM AKST by NWS Anchorage AK\",\n                \"description\": \"Coastal Waters Forecast for the Northern Gulf of Alaska Coast\\nup to 100 nm out including Kodiak Island and Cook Inlet.\\n\\nWind forecasts reflect the predominant speed and direction\\nexpected. Sea forecasts represent an average of the highest\\none-third of the combined wind wave and swell height.\\n\\n.TODAY...E wind 25 kt becoming SE 15 kt in the afternoon.\\nSeas 5 ft subsiding to 3 ft in the afternoon. Rain.\\n.TONIGHT...S wind 15 kt. Seas 3 ft.\\n.THU...E wind 15 kt. Seas 3 ft.\\n.THU NIGHT...NE wind 15 kt. Seas 3 ft.\\n.FRI...N wind 25 kt. Seas 5 ft.\\n.SAT THROUGH SUN...N wind 30 kt. Seas 7 ft.\",\n                \"instruction\": null,\n                \"response\": \"Avoid\",\n                \"parameters\": {\n                    \"AWIPSidentifier\": [\n                        \"CWFAER\"\n                    ],\n                    \"WMOidentifier\": [\n                        \"FZAK51 PAFC 031302\"\n                    ],\n                    \"NWSheadline\": [\n                        \"SMALL CRAFT ADVISORY TODAY\"\n                    ],\n                    \"BLOCKCHANNEL\": [\n                        \"EAS\",\n                        \"NWEM\",\n                        \"CMAS\"\n                    ],\n                    \"VTEC\": [\n                        \"/O.NEW.PAFC.SC.Y.9738.251203T1400Z-251204T0200Z/\"\n                    ],\n                    \"eventEndingTime\": [\n                        \"2025-12-03T17:00:00-09:00\"\n                    ]\n                },\n                \"scope\": \"Public\",\n                \"code\": \"IPAWSv1.0\",\n                \"language\": \"en-US\",\n                \"web\": \"http://www.weather.gov\",\n                \"eventCode\": {\n                    \"SAME\": [\n                        \"NWS\"\n                    ],\n                    \"NationalWeatherService\": [\n                        \"SCY\"\n                    ]\n                }\n            }\n        },\n        {\n            \"id\": \"https://api.weather.gov/alerts/urn:oid:2.49.0.1.840.0.3fac73b358a1e250101ceb2ba749b5bee3a29f80.003.1\",\n            \"type\": \"Feature\",\n            \"geometry\": null,\n            \"properties\": {\n                \"@id\": \"https://api.weather.gov/alerts/urn:oid:2.49.0.1.840.0.3fac73b358a1e250101ceb2ba749b5bee3a29f80.003.1\",\n                \"@type\": \"wx:Alert\",\n                \"id\": \"urn:oid:2.49.0.1.840.0.3fac73b358a1e250101ceb2ba749b5bee3a29f80.003.1\",\n                \"areaDesc\": \"Gravel Point to Cape Cleare out to 15 NM\",\n                \"geocode\": {\n                    \"SAME\": [\n                        \"058711\"\n                    ],\n                    \"UGC\": [\n                        \"PKZ711\"\n                    ]\n                },\n                \"affectedZones\": [\n                    \"https://api.weather.gov/zones/forecast/PKZ711\"\n                ],\n                \"references\": [],\n                \"sent\": \"2025-12-03T04:02:00-09:00\",\n                \"effective\": \"2025-12-03T04:02:00-09:00\",\n                \"onset\": \"2025-12-03T04:00:00-09:00\",\n                \"expires\": \"2025-12-03T16:30:00-09:00\",\n                \"ends\": \"2025-12-04T17:00:00-09:00\",\n                \"status\": \"Actual\",\n                \"messageType\": \"Alert\",\n                \"category\": \"Met\",\n                \"severity\": \"Minor\",\n                \"certainty\": \"Likely\",\n                \"urgency\": \"Expected\",\n                \"event\": \"Small Craft Advisory\",\n                \"sender\": \"w-nws.webmaster@noaa.gov\",\n                \"senderName\": \"NWS Anchorage AK\",\n                \"headline\": \"Small Craft Advisory issued December 3 at 4:02AM AKST until December 4 at 5:00PM AKST by NWS Anchorage AK\",\n                \"description\": \"Coastal Waters Forecast for the Northern Gulf of Alaska Coast\\nup to 100 nm out including Kodiak Island and Cook Inlet.\\n\\nWind forecasts reflect the predominant speed and direction\\nexpected. Sea forecasts represent an average of the highest\\none-third of the combined wind wave and swell height.\\n\\n.TODAY...SE wind 20 kt in the morning becoming variable 10 kt.\\nSeas 10 ft.\\n.TONIGHT...Variable wind 10 kt. Seas 9 ft.\\n.THU...Variable wind 10 kt. Seas 8 ft.\\n.THU NIGHT...Variable wind 10 kt. Seas 6 ft.\\n.FRI...NE wind 15 kt. Seas 5 ft.\\n.SAT THROUGH SUN...NE wind 30 kt. Seas 9 ft.\",\n                \"instruction\": null,\n                \"response\": \"Avoid\",\n                \"parameters\": {\n                    \"AWIPSidentifier\": [\n                        \"CWFAER\"\n                    ],\n                    \"WMOidentifier\": [\n                        \"FZAK51 PAFC 031302\"\n                    ],\n                    \"NWSheadline\": [\n                        \"SMALL CRAFT ADVISORY THROUGH THURSDAY\"\n                    ],\n                    \"BLOCKCHANNEL\": [\n                        \"EAS\",\n                        \"NWEM\",\n                        \"CMAS\"\n                    ],\n                    \"VTEC\": [\n                        \"/O.NEW.PAFC.SC.Y.9731.251203T1300Z-251205T0200Z/\"\n                    ],\n                    \"eventEndingTime\": [\n                        \"2025-12-04T17:00:00-09:00\"\n                    ]\n                },\n                \"scope\": \"Public\",\n                \"code\": \"IPAWSv1.0\",\n                \"language\": \"en-US\",\n                \"web\": \"http://www.weather.gov\",\n                \"eventCode\": {\n                    \"SAME\": [\n                        \"NWS\"\n                    ],\n                    \"NationalWeatherService\": [\n                        \"SCY\"\n                    ]\n                }\n            }\n        },\n        {\n            \"id\": \"https://api.weather.gov/alerts/urn:oid:2.49.0.1.840.0.3fac73b358a1e250101ceb2ba749b5bee3a29f80.019.1\",\n            \"type\": \"Feature\",\n            \"geometry\": null,\n            \"properties\": {\n                \"@id\": \"https://api.weather.gov/alerts/urn:oid:2.49.0.1.840.0.3fac73b358a1e250101ceb2ba749b5bee3a29f80.019.1\",\n                \"@type\": \"wx:Alert\",\n                \"id\": \"urn:oid:2.49.0.1.840.0.3fac73b358a1e250101ceb2ba749b5bee3a29f80.019.1\",\n                \"areaDesc\": \"Marmot Island To Sitkinak from 15 to 85 NM\",\n                \"geocode\": {\n                    \"SAME\": [\n                        \"058734\"\n                    ],\n                    \"UGC\": [\n                        \"PKZ734\"\n                    ]\n                },\n                \"affectedZones\": [\n                    \"https://api.weather.gov/zones/forecast/PKZ734\"\n                ],\n                \"references\": [],\n                \"sent\": \"2025-12-03T04:02:00-09:00\",\n                \"effective\": \"2025-12-03T04:02:00-09:00\",\n                \"onset\": \"2025-12-03T04:00:00-09:00\",\n                \"expires\": \"2025-12-03T16:30:00-09:00\",\n                \"ends\": \"2025-12-04T17:00:00-09:00\",\n                \"status\": \"Actual\",\n                \"messageType\": \"Alert\",\n                \"category\": \"Met\",\n                \"severity\": \"Minor\",\n                \"certainty\": \"Likely\",\n                \"urgency\": \"Expected\",\n                \"event\": \"Small Craft Advisory\",\n                \"sender\": \"w-nws.webmaster@noaa.gov\",\n                \"senderName\": \"NWS Anchorage AK\",\n                \"headline\": \"Small Craft Advisory issued December 3 at 4:02AM AKST until December 4 at 5:00PM AKST by NWS Anchorage AK\",\n                \"description\": \"Coastal Waters Forecast for the Northern Gulf of Alaska Coast\\nup to 100 nm out including Kodiak Island and Cook Inlet.\\n\\nWind forecasts reflect the predominant speed and direction\\nexpected. Sea forecasts represent an average of the highest\\none-third of the combined wind wave and swell height.\\n\\n.TODAY...S wind 20 kt. Seas 13 ft.\\n.TONIGHT...S wind 15 kt. Seas 11 ft.\\n.THU...SE wind 15 kt. Seas 10 ft.\\n.THU NIGHT...NE wind 15 kt. Seas 8 ft.\\n.FRI THROUGH SAT...NW wind 25 kt. Seas 9 ft.\\n.SUN...NW wind 25 kt. Seas 13 ft.\",\n                \"instruction\": null,\n                \"response\": \"Avoid\",\n                \"parameters\": {\n                    \"AWIPSidentifier\": [\n                        \"CWFAER\"\n                    ],\n                    \"WMOidentifier\": [\n                        \"FZAK51 PAFC 031302\"\n                    ],\n                    \"NWSheadline\": [\n                        \"SMALL CRAFT ADVISORY THROUGH THURSDAY\"\n                    ],\n                    \"BLOCKCHANNEL\": [\n                        \"EAS\",\n                        \"NWEM\",\n                        \"CMAS\"\n                    ],\n                    \"VTEC\": [\n                        \"/O.NEW.PAFC.SC.Y.9737.251203T1300Z-251205T0200Z/\"\n                    ],\n                    \"eventEndingTime\": [\n                        \"2025-12-04T17:00:00-09:00\"\n                    ]\n                },\n                \"scope\": \"Public\",\n                \"code\": \"IPAWSv1.0\",\n                \"language\": \"en-US\",\n                \"web\": \"http://www.weather.gov\",\n                \"eventCode\": {\n                    \"SAME\": [\n                        \"NWS\"\n                    ],\n                    \"NationalWeatherService\": [\n                        \"SCY\"\n                    ]\n                }\n            }\n        },\n        {\n            \"id\": \"https://api.weather.gov/alerts/urn:oid:2.49.0.1.840.0.3fac73b358a1e250101ceb2ba749b5bee3a29f80.005.1\",\n            \"type\": \"Feature\",\n            \"geometry\": null,\n    
